vi "OpenScan-packed DRAM-FPGA.vi"() -> ()   [LabVIEW 2015]
uses:
  <vilib>/rvi/Emulation/niFpgaGetClockAttributes.vi
  <vilib>/rvi/Emulation/niFpgaSctlEmulationGetInTimedLoop.vi
  <vilib>/rvi/Emulation/niFpgaEmulationReportErrorSimple.vi
  Globals/Global_Sample per Frame.vi
  <vilib>/rvi/Emulation/niFpgaCriticalErrorInLSC.vi
  <vilib>/rvi/Emulation/niFpgaProcessEmulError.vi
  Globals/Global Variable_Pixel Clock.vi
panel:
  out "Waiting?":bool
  out "Stopping?":bool
  out "FPGA stop":bool
  out "FPGA loop count":i32
  out "Frame address_indicator":u32
  out "Scanning?":bool
  in  "Ready to Scan":bool
  in  "Frame number":i32
  out "Frame waveform output finish?":bool
  out "Frame acquisition finish?":bool
  out "loop count":i32
  out "Display_frames done":i32
  out "Averaged data address":u32
  out "Frame imaging data averaged?":bool
  out "Averaged image displayed?":bool
  in  "Kalman gain":fxp<+,16,1>=0.1015625
  in  "Filter gain":fxp<+,16,0>=0.8000030517578125
  out "Pixel clock (Indicator)":bool
  out "Image averaging done?":bool
  out "Data":u32
  out "Galvo signal readed":u32
  out "Request address":u32
  out "Line clock":bool
  in  "Pixel clock_pulse width(tick)":i32
  in  "Resolution":i32
  in  "Pixel pulse_initial delay":i32
  in  "Frame retrace time":u32 caption="Frame retrace time (ms)"
  in  "Num of undershoot":i32
  in  "Elements per line":i32
  in  "Num of elements":u32
  in  "Pixel time (tick)":i32
  out "Write DRAM done?":bool
  in  "Total elements":u32
  out "Frame Galvo signal write done?":bool
  in  "max addr":u32=1024
  in  "Write DRAM enable?":bool
  in  "Write Frame Galvo signal?":bool
  out "Imaging data unpacked for Kalman":u32
  out "Max DRAM address _indicator":u32
  out "Imaging data averaged":u32
  out "Imaging data DRAM address":u32
  out "Number of frames indicator":i32
  out "Waveform output loop count_indicator":i32
  out "Num of elements_indicator":u32=512000
  out "Frame address_Global":u32
  out "Frams done_indicator":i32
  out "Num of data":u32
  out "Kalman Imaging data address":u32
  out "Display imaging data address":u32
  out "Galvo signal readed_indicator":u32
  out "Samples acquired":u32
  out "Samples per frame_Global":u32
  out "image data address indicator":u32
  out "Address counter":u32
  out "Pixel clock_indicator":bool
  out "Averaged image displayed? _indicator":bool
  out "Data indicator":u32
  in  "Max DRAM address":u32
  in  "Number of frames":i32
  in  "Samples per frame control":u32=262144
  # "Running Status"
  # "Waveform Data Loading"
  # "Photon Counting"
  # "Imaging Data Display"
  # "Waveform Generation"
  # "Controller"
  # "Indicator"
  # "Debug Indicators"
  # "Initialization"
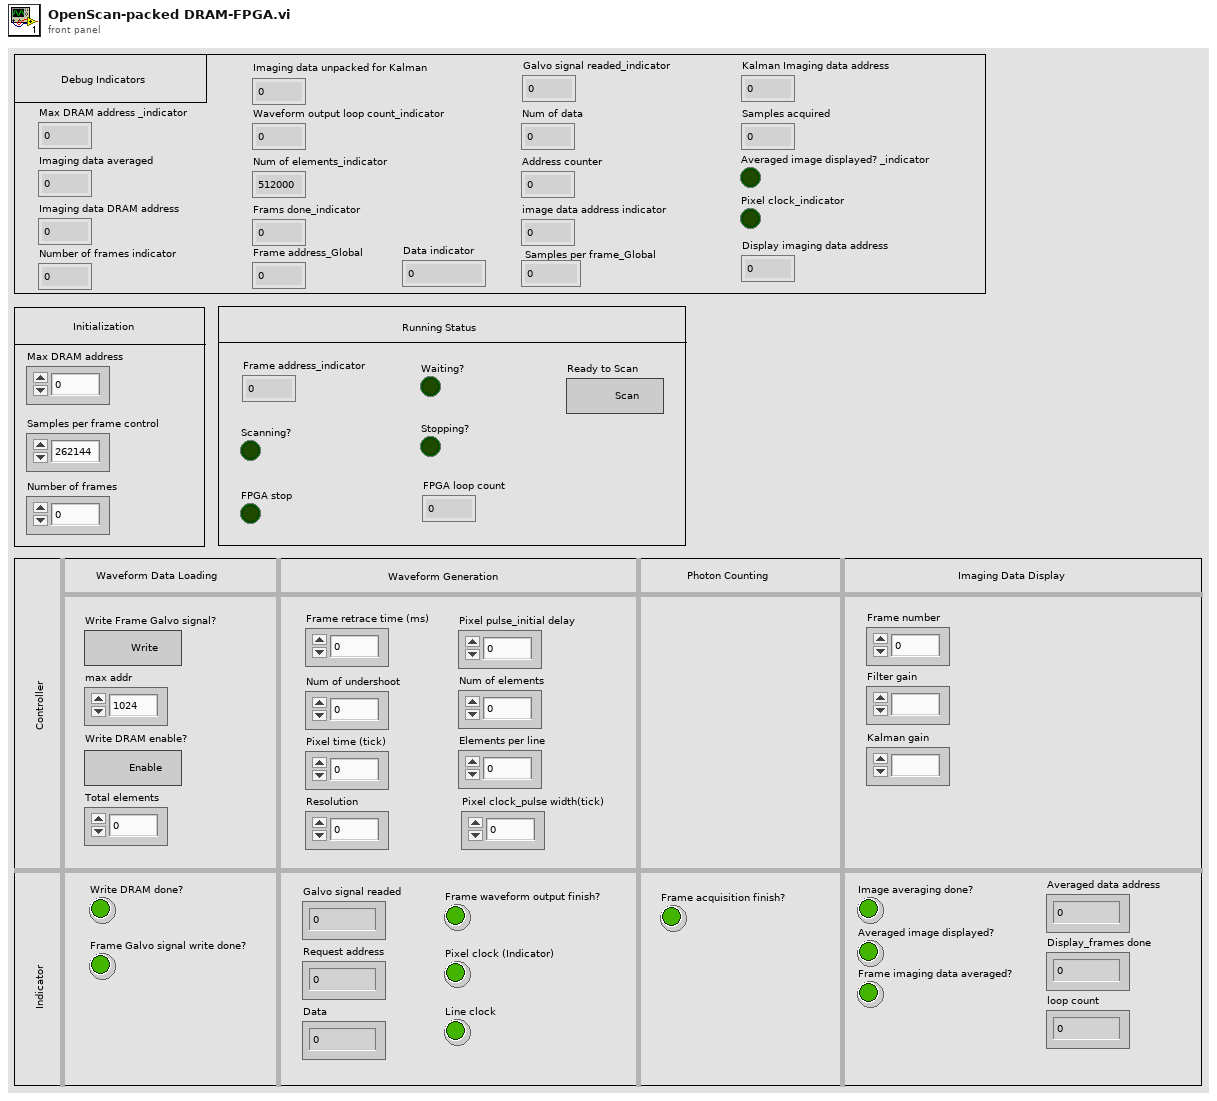
[diagram p1: front panel]
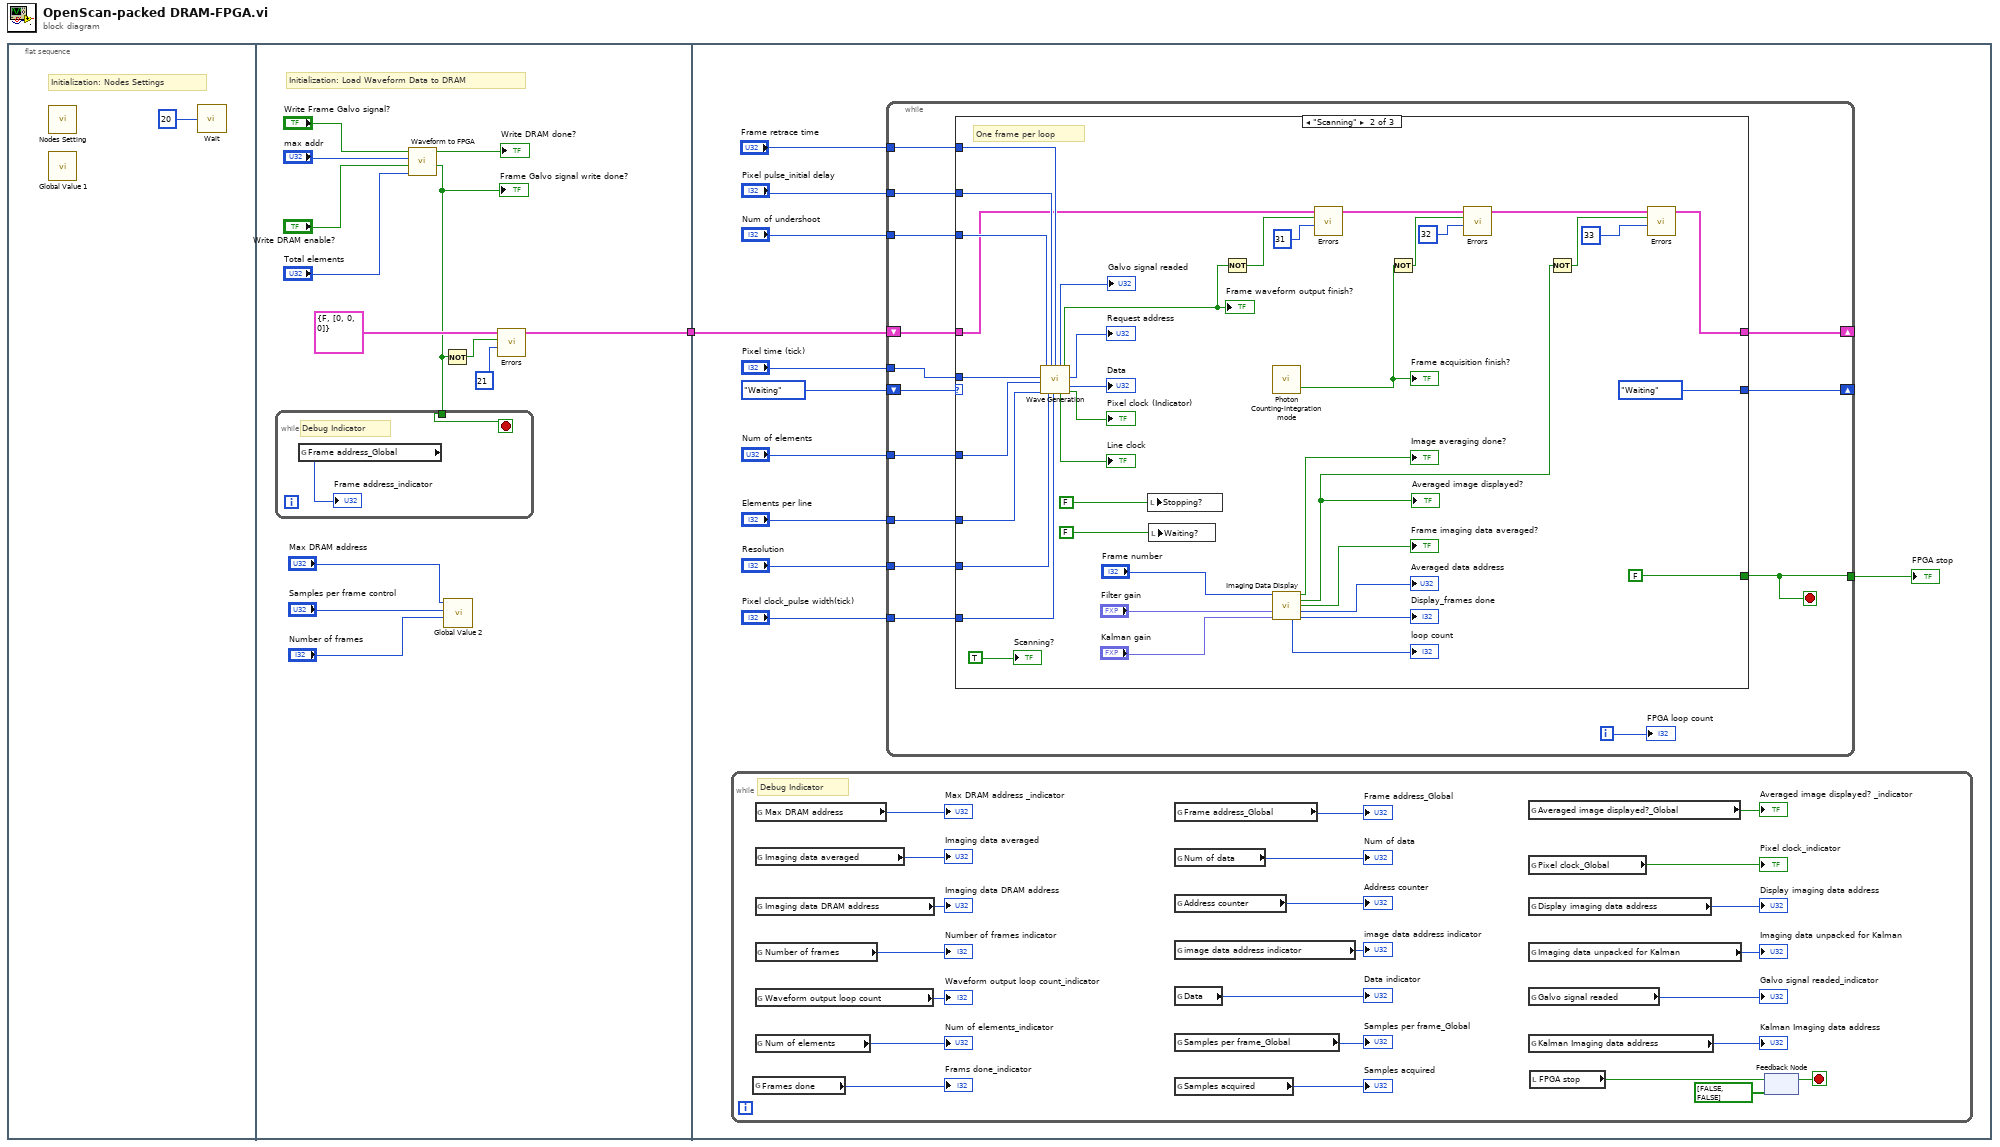
[diagram p0: block diagram]
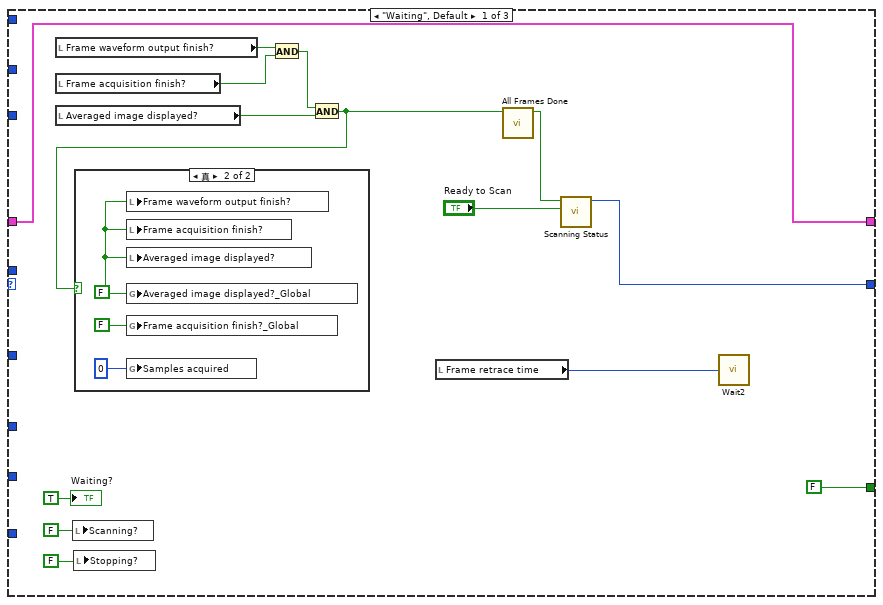
[diagram p2: hidden frame]
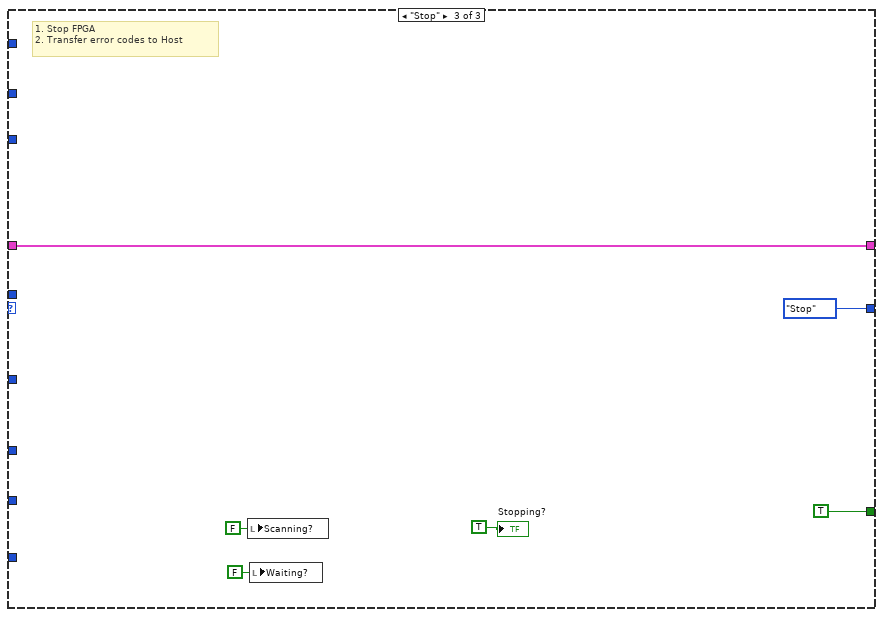
[diagram p4: hidden frame]
diagram:
  n1 = flat-sequence {
    tunnel: [w4] -> w1
    tunnel: w1 -> [w18]
    frame #0 {
      # "Initialization: Nodes Settings"
      n2 = call "Nodes Setting.vi"() -> ()  [unwired: 12 in]
      n3 = call "Global Value 1.vi"() -> ()  [unwired: 12 in]
      n4 = call "Wait"("Count(mSec)"=u32 20) -> ()  [unwired: 1 out]
    }
    frame #1 {
      # "Initialization: Load Waveform Data to DRAM"
      n5 = call "Waveform to FPGA.vi"("Write Frame Galvo signal?"="Write Frame Galvo signal?", "max addr"="max addr", "Write DRAM enable?"="Write DRAM enable?", "Total elements"="Total elements") -> ("Write DRAM done?"=→"Write DRAM done?":bool, "Frame Galvo signal write done?"=w6:bool)  [unwired: 5 in]
      "Frame Galvo signal write done?" <- w6
      n6 = while {
        tunnel: w6 -> [w16]
        stop <- w16 stop-if-true
        # "Debug Indicator"
        n7 = global read "Global_Sample per Frame.vi" "Frame address_Global"() -> (→"Frame address_indicator":u32)
      }
      n8 = Not(x=w6) -> (.not. x?=w5:bool)
      n9 = call "Global Value 2.vi"("Number of frames"="Number of frames", "Samples per frame control"="Samples per frame control", "Max DRAM address"="Max DRAM address") -> ()  [unwired: 9 in]
      n10 = call "Errors.vi"("Error Codes"=u16 21, "Status"=w5, "Error in"=cluster{"status":bool, "Codes":u16[]} {"status"=FALSE, "Codes"=[0, 0, 0]}) -> ("Error out"=w4:cluster{"status":bool, "Codes":u16[]})  [unwired: 7 in, 1 out]
    }
    frame #2 {
      n11 = while {
        stop <- w37 stop-if-true
        # "Debug Indicator"
        n12 = global read "Global_Sample per Frame.vi" "Frames done"() -> (→"Frams done_indicator":i32)
        n13 = global read "Global_Sample per Frame.vi" "Max DRAM address"() -> (→"Max DRAM address _indicator":u32)
        n14 = global read "Global_Sample per Frame.vi" "Imaging data averaged"() -> (→"Imaging data averaged":u32)
        n15 = global read "Global_Sample per Frame.vi" "Imaging data DRAM address"() -> (→"Imaging data DRAM address":u32)
        n16 = global read "Global_Sample per Frame.vi" "Number of frames"() -> (→"Number of frames indicator":i32)
        n17 = global read "Global_Sample per Frame.vi" "Waveform output loop count"() -> (→"Waveform output loop count_indicator":i32)
        n18 = global read "Global_Sample per Frame.vi" "Num of elements"() -> (→"Num of elements_indicator":u32)
        n19 = global read "Global_Sample per Frame.vi" "Frame address_Global"() -> (→"Frame address_Global":u32)
        n20 = global read "Global_Sample per Frame.vi" "Num of data"() -> (→"Num of data":u32)
        n21 = global read "Global_Sample per Frame.vi" "Address counter"() -> (→"Address counter":u32)
        n22 = global read "Global_Sample per Frame.vi" "image data address indicator"() -> (→"image data address indicator":u32)
        n23 = global read "Global_Sample per Frame.vi" "Data"() -> (→"Data indicator":u32)
        n24 = global read "Global_Sample per Frame.vi" "Samples per frame_Global"() -> (→"Samples per frame_Global":u32)
        n25 = global read "Global_Sample per Frame.vi" "Samples acquired"() -> (→"Samples acquired":u32)
        n26 = global read "Global_Sample per Frame.vi" "Averaged image displayed?_Global"() -> (→"Averaged image displayed? _indicator":bool)
        n27 = global read "Global Variable_Pixel Clock.vi" "Pixel clock_Global"() -> (→"Pixel clock_indicator":bool)
        n28 = global read "Global_Sample per Frame.vi" "Display imaging data address"() -> (→"Display imaging data address":u32)
        n29 = global read "Global_Sample per Frame.vi" "Imaging data unpacked for Kalman"() -> (→"Imaging data unpacked for Kalman":u32)
        n30 = global read "Global_Sample per Frame.vi" "Galvo signal readed"() -> (→"Galvo signal readed_indicator":u32)
        n31 = global read "Global_Sample per Frame.vi" "Kalman Imaging data address"() -> (→"Kalman Imaging data address":u32)
        n32 = local read "FPGA stop"() -> (w40:bool)
        n33 = feedback-in #1(w40) -> ()
        n34 = feedback #1(bool[] [FALSE, FALSE]) -> (w37:bool)
      }
      n35 = while {
        shift-right: [w64] -> _
        shift-left: enum16{"Waiting", "Scanning", "Stop"}."Waiting" -> [w65]
        shift-right: [w52] -> _
        shift-left: w18 -> [w53]
        tunnel: "Frame retrace time" -> [w63]
        tunnel: "Pixel pulse_initial delay" -> [w62]
        tunnel: "Num of undershoot" -> [w61]
        tunnel: "Pixel time (tick)" -> [w60]
        tunnel: "Num of elements" -> [w59]
        tunnel: "Elements per line" -> [w58]
        tunnel: "Resolution" -> [w57]
        tunnel: "Pixel clock_pulse width(tick)" -> [w56]
        tunnel: [w54] -> w19
        i -> [w55]
        stop <- w54 stop-if-true
        n36 = case shown="\"Scanning\"" w65 {
          tunnel: [w78 enum16{"Waiting", "Scanning", "Stop"}."Waiting" enum16{"Waiting", "Scanning", "Stop"}."Stop"] -> w64
          tunnel: w53 -> [w79 w95 w127]
          tunnel: [w79 w85 w127] -> w52
          tunnel: w63 -> [_ w110 _]
          tunnel: w62 -> [_ w109 _]
          tunnel: w61 -> [_ w108 _]
          tunnel: w60 -> [_ w107 _]
          tunnel: w59 -> [_ w106 _]
          tunnel: w58 -> [_ w105 _]
          tunnel: w57 -> [_ w104 _]
          tunnel: w56 -> [_ w103 _]
          tunnel: [FALSE FALSE TRUE] -> w54
          frame "Waiting", Default {
            n37 = local read "Frame waveform output finish?"() -> (w72:bool)
            n38 = local read "Frame acquisition finish?"() -> (w73:bool)
            n39 = local read "Averaged image displayed?"() -> (w74:bool)
            n40 = local write "Scanning?"(FALSE ("Scanning?")) -> ()
            n41 = local write "Stopping?"(FALSE ("Stopping?")) -> ()
            n42 = And(x=w72, y=w73) -> (x .and. y?=w75:bool)
            n43 = And(x=w75, y=w74) -> (x .and. y?=w69:bool)
            n44 = case shown="真" w69 {
              frame False {
              }
              frame True {
                w80 = FALSE ("Averaged image displayed?")
                n45 = local write "Frame waveform output finish?"(w80) -> ()
                n46 = local write "Frame acquisition finish?"(w80) -> ()
                n47 = local write "Averaged image displayed?"(w80) -> ()
                n48 = global write "Global_Sample per Frame.vi" "Averaged image displayed?_Global"(w80) -> ()
                n49 = global write "Global_Sample per Frame.vi" "Frame acquisition finish?_Global"(FALSE ("Frame acquisition finish?")) -> ()
                n50 = global write "Global_Sample per Frame.vi" "Samples acquired"(u32 0 ("Frame address")) -> ()
              }
            }
            n51 = local read "Frame retrace time"() -> (w70:u32)
            n52 = call "All Frames Done.vi"("Done in"=w69) -> ("Done out"=w71:bool)  [unwired: 10 in]
            n53 = call "Scanning Status.vi"("Ready to Scan"="Ready to Scan", "Done out"=w71) -> ("Status out"=w78:enum16{"Waiting", "Scanning", "Stop"})  [unwired: 9 in]
            n54 = call "Wait2"("Count(mSec)"=w70) -> ()  [unwired: 1 out]
            "Waiting?" <- TRUE
          }
          frame "Scanning" {
            # "One frame per loop"
            n55 = call "Wave Generation.vi"("Pixel time (tick)"=w107, "Num of elements"=w106, "Elements per line"=w105, "Num of undershoot"=w108, "Resolution"=w104, "Pixel pulse_initial delay"=w109, "Pixel clock_pulse width(tick)"=w103, "Frame retrace time"=w110) -> ("Frame waveform output finish?"=w94:bool, "Line clock"=→"Line clock":bool, "Request address"=→"Request address":u32, "Galvo signal readed"=→"Galvo signal readed":u32, "Data"=→"Data":u32, "Pixel clock"=→"Pixel clock (Indicator)":bool)  [unwired: 6 in]
            "Frame waveform output finish?" <- w94
            n56 = local write "Stopping?"(FALSE ("Stopping?")) -> ()
            n57 = local write "Waiting?"(FALSE ("Waiting?")) -> ()
            n58 = Not(x=w94) -> (.not. x?=w93:bool)
            n59 = call "Photon Counting-integration mode.vi"() -> ("Frame acquisition finish?"=w90:bool)  [unwired: 19 in]
            "Frame acquisition finish?" <- w90
            n60 = call "Imaging Data Display.vi"("Frame number"="Frame number", "Filter gain"="Filter gain", "Kalman gain"="Kalman gain") -> ("Image averaging done?"=→"Image averaging done?":bool, "Averaged image displayed?"=w87:bool, "Frame imaging data Averaged?"=→"Frame imaging data averaged?":bool, "Averaged data address"=→"Averaged data address":u32, "loop count"=→"loop count":i32, "Display_frames done"=→"Display_frames done":i32)  [unwired: 7 in]
            "Averaged image displayed?" <- w87
            n61 = call "Errors.vi"("Error Codes"=u16 31, "Status"=w93, "Error in"=w95) -> ("Error out"=w91:cluster{"status":bool, "Codes":u16[]})  [unwired: 7 in, 1 out]
            n62 = Not(x=w90) -> (.not. x?=w84:bool)
            n63 = call "Errors.vi"("Error Codes"=u16 32, "Status"=w84, "Error in"=w91) -> ("Error out"=w88:cluster{"status":bool, "Codes":u16[]})  [unwired: 7 in, 1 out]
            n64 = Not(x=w87) -> (.not. x?=w83:bool)
            n65 = call "Errors.vi"("Error Codes"=u16 33, "Status"=w83, "Error in"=w88) -> ("Error out"=w85:cluster{"status":bool, "Codes":u16[]})  [unwired: 7 in, 1 out]
            "Scanning?" <- TRUE
          }
          frame "Stop" {
            # "1. Stop FPGA\n2. Transfer error codes to Host"
            n66 = local write "Scanning?"(FALSE ("Scanning?")) -> ()
            n67 = local write "Waiting?"(FALSE ("Waiting?")) -> ()
            "Stopping?" <- TRUE
          }
        }
        "FPGA loop count" <- w55
      }
      "FPGA stop" <- w19
    }
  }
